vi "HexStringToI32.vi"(0 "Input String":string, 7 "Starting Offset":i32) -> (4 "Number Out":i32)   [LabVIEW 2016]
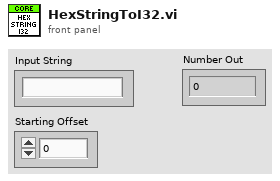
[diagram p1: front panel]
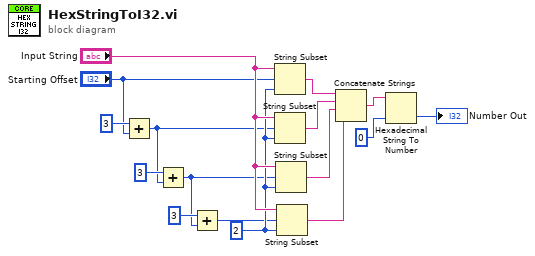
[diagram p0: block diagram]
diagram:
  w8 = 2 ("offset (0)")
  n1 = Add(x=3, y="Starting Offset") -> (x+y=w3:i32)
  n2 = Add(x=3, y=w3) -> (x+y=w1:i32)
  n3 = Add(x=3, y=w1) -> (x+y=w2:i32)
  n4 = String Subset(string="Input String", offset (0)="Starting Offset", length (rest)=w8) -> (substring=w14:string)
  n5 = String Subset(string="Input String", offset (0)=w3, length (rest)=w8) -> (substring=w10:string)
  n6 = String Subset(string="Input String", offset (0)=w1, length (rest)=w8) -> (substring=w6:string)
  n7 = String Subset(string="Input String", offset (0)=w2, length (rest)=w8) -> (substring=w5:string)
  n8 = Concatenate Strings(w14, w10, w6, w5) -> (w16:string)
  n9 = Hexadecimal String To Number(string=w16, default (0uL)=0) -> (number=→"Number Out":i32)  [unwired: 1 in, 1 out]
